vi "CTL_PumpController.vi"(7 "Pump CtlRef In":T1, 8 "Input cluster":cluster{"Spec HI in":dbl, "Spec Lo in":dbl}, 9 "BinSearch":bool, 10 "Res Switched?":bool, 11 "Level PV":dbl) -> (2 "PV Out":dbl, 3 "PumpCTLOutput":T2 {"PV" scale=0.0..10.0})   [LabVIEW 2024]
uses:
  Control Definitions/Def PumpCtlOutputs.ctl
  Control Definitions/Def PumpCtlRefs.ctl
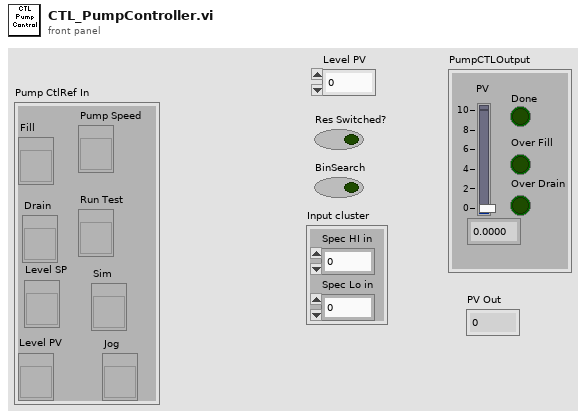
[diagram p1: front panel]
types:
  T1 = typedef "Def PumpCtlRefs.ctl" = cluster{"Fill ":refnum<vi>, "Drain":refnum<vi>, "Level PV":refnum<vi>, "Pump Speed":refnum<vi>, "Run Test":refnum<vi>, "Sim":refnum<vi>, "Jog":refnum<vi>, "Level SP":refnum<vi>}
  T2 = typedef "Def PumpCtlOutputs.ctl" = cluster{"PV":dbl, "Done":bool, "Over Fill":bool, "Over Drain":bool}
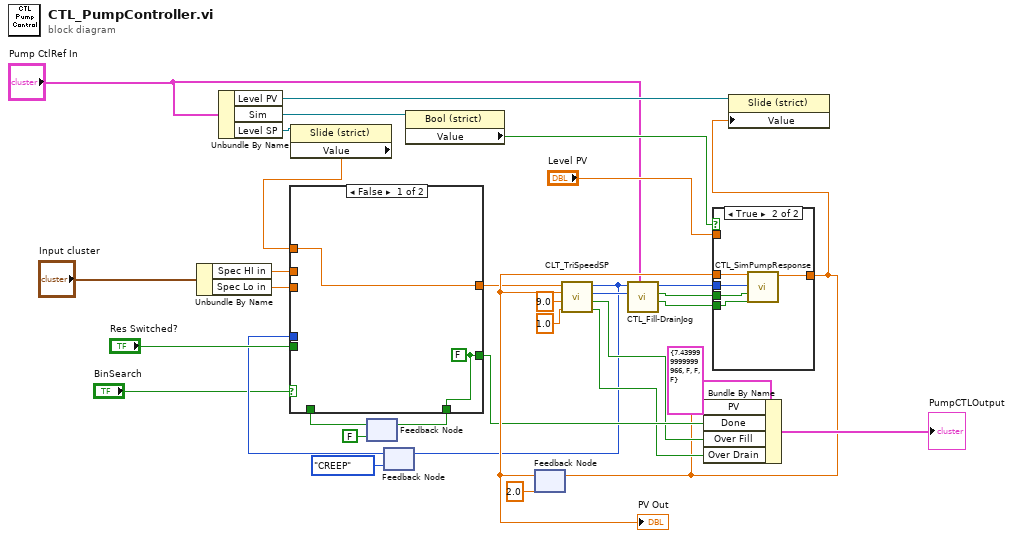
[diagram p0: block diagram]
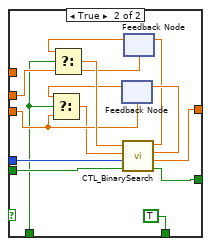
[diagram p2: hidden frame]
diagram:
  n1 = Unbundle By Name("Input cluster") -> ("Spec HI in"=w31:dbl, "Spec Lo in"=w32:dbl)
  n2 = Unbundle By Name("Pump CtlRef In") -> ("Level PV"=w16:refnum<vi>, "Sim"=w18:refnum<vi>, "Level SP"=w19:refnum<vi>)
  n3 = property class="Slide (strict)"(reference=w19) -> ("Value"=w20:dbl)  [unwired: 1 in, 2 out]
  n4 = feedback #1(FALSE) -> (w2:bool)
  n5 = feedback #2(enum16{"FAST", "SLOW", "CREEP", "STOP"}."CREEP" ("Pump Speed")) -> (w8:enum16{"FAST", "SLOW", "CREEP", "STOP"})
  n6 = case shown="False" "BinSearch" {
    tunnel: w31 -> [_ w41]
    tunnel: w32 -> [_ w39]
    tunnel: [w35 w48] -> w21
    tunnel: w20 -> [w35 _]
    tunnel: "Res Switched?" -> [_ w49]
    tunnel: [w34 w47] -> w25
    tunnel: w8 -> [_ w44]
    tunnel: [w34 TRUE] -> w3
    tunnel: w2 -> [_ w36]
    frame False {
      w34 = FALSE ("Done")
    }
    frame True {
      n7 = feedback #3(w39) -> (w40:dbl)
      n8 = Select(t=w40, s=w36, f=w39) -> (s? t:f=w38:dbl)
      n9 = feedback #4(w41) -> (w43:dbl)
      n10 = Select(t=w43, s=w36, f=w41) -> (s? t:f=w42:dbl)
      n11 = call "CTL_BinarySearch.vi"("Switched?"=w49, "PumpSpeed"=w44, "Spec Lo in"=w38, "Spec HI in"=w42) -> ("Done"=w47:bool, "Guess"=w48:dbl, "Spec Lo out"=w46:dbl, "Spec HI out"=w45:dbl)  [unwired: 4 in]
      n12 = feedback-in #3(w46) -> ()
      n13 = feedback-in #4(w45) -> ()
    }
  }
  n14 = feedback-in #1(w3) -> ()
  n15 = property class="Bool (strict)"(reference=w18) -> ("Value"=w28:bool)  [unwired: 1 in, 2 out]
  n16 = feedback #5(2.0 ("PV Out")) -> (w29:dbl)
  "PV Out" <- w29
  n17 = call "CLT_TriSpeedSP.vi"("Empty in"=1.0, "Full in"=9.0, "Level PV"=w29, "Level SP"=w21) -> ("OverDrain"=w24:bool, "OverFill"=w23:bool, "Pump Direction"=w11:enum16{"FILL", "DRAIN"}, "Pump Speed"=w10:enum16{"FAST", "SLOW", "CREEP", "STOP"})  [unwired: 4 in]
  n18 = feedback-in #2(w10) -> ()
  n19 = call "CTL_Fill-DrainJog.vi"("Pump CtlRef In"="Pump CtlRef In", "Pump Direction"=w11, "Pump Speed"=w10) -> ("Drain Out"=w14:bool, "Fill Out"=w13:bool, "Pump Speed Out"=w12:enum16{"FAST", "SLOW", "CREEP", "STOP"})  [unwired: 4 in, 2 out]
  n20 = case shown="True" w28 {
    tunnel: w29 -> [_ w55]
    tunnel: [w50 w54] -> w22
    tunnel: "Level PV" -> [w50 _]
    tunnel: w12 -> [_ w53]
    tunnel: w13 -> [_ w52]
    tunnel: w14 -> [_ w51]
    frame False {
    }
    frame True {
      n21 = call "CTL_SimPumpResponse.vi"("Drain"=w51, "Fill"=w52, "Pump Speed"=w53, "PV IN"=w55) -> ("PV Out"=w54:dbl)  [unwired: 7 in]
    }
  }
  n22 = feedback-in #5(w22) -> ()
  n23 = Bundle By Name(cluster=T2 {"PV"=7.439999999999966, "Done"=FALSE, "Over Fill"=FALSE, "Over Drain"=FALSE} ("PumpCTLOutput"), "PV"=w22, "Done"=w25, "Over Fill"=w23, "Over Drain"=w24) -> (→"PumpCTLOutput":T2)
  n24 = property class="Slide (strict)"(reference=w16, "Value"=w22) -> ()  [unwired: 1 in, 2 out]
